vi "Copy_Files.vi"(8 "error in (no error)":errorcluster, 11 "Build in":refnum<class "AB_DLL.lvclass">) -> (0 "error out":errorcluster, 3 "Build out":refnum<class "AB_DLL.lvclass">)   [LabVIEW 2020, in "AB_DLL.lvclass"]
uses:
  <vilib>/AppBuilder/AB_Classes/DLL/AB_DLL.lvclass
  e:/builds/penguin/labview/branches/2020/dev/dist/vi.lib/AppBuilder/AB_Classes/TargetFile/AB_Targetfile.lvclass
  <vilib>/AppBuilder/AB_Classes/DLL/AB_DLL.lvclass/AB_DLL.ctl
  <vilib>/AppBuilder/AB_Classes/Application/AB_Application.lvclass
  <vilib>/AppBuilder/AB_Classes/TargetFile/AB_Targetfile.lvclass
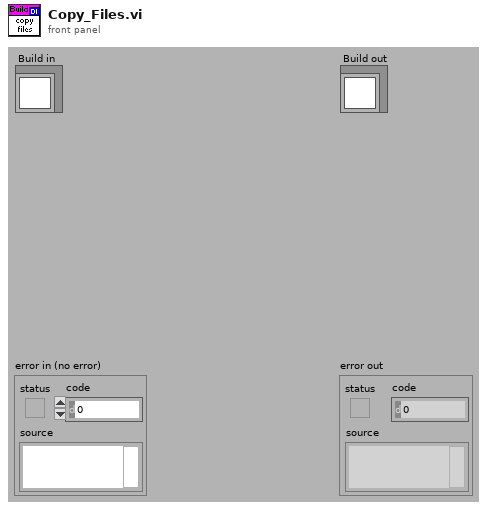
[diagram p1: front panel]
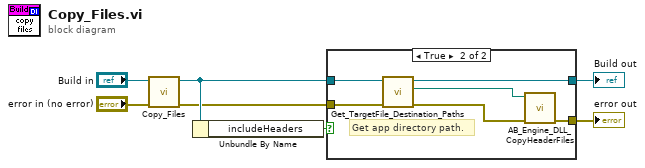
[diagram p0: block diagram]
diagram:
  n1 = call-parent "Copy_Files.vi"("error in (no error)"="error in (no error)", "Build in"="Build in") -> ("error out"=w1:errorcluster, "Build out"=w3:refnum<class "AB_DLL.lvclass">)  [unwired: 8 out]
  n2 = Unbundle By Name(w3) -> ("includeHeaders"=w4:bool)
  n3 = case shown="True" w4 {
    tunnel: [w8 w15] -> w5
    tunnel: w3 -> [w9 w12]
    tunnel: [w9 w14] -> w2
    tunnel: w1 -> [w8 w11]
    frame False {
    }
    frame True {
      # "Get app directory path."
      n4 = call <vilib>:"Get_TargetFile_Destination_Paths.vi"("error in (no error)"=w11, "AB_Targetfile in"=w12) -> ("error out"=w10:errorcluster, "destination path"=w13:path, "AB_Targetfile out"=w14:refnum<class "AB_DLL.lvclass">)  [unwired: 7 out]
      n5 = call <vilib>:"AB_Engine_DLL_CopyHeaderFiles.vi"("error in (no error)"=w10, "Path"=w13) -> ("error out"=w15:errorcluster)  [unwired: 1 in, 8 out]
    }
  }
  "error out" <- w5
  "Build out" <- w2
